vi "Compression_Simulation_Get Target Measurements.vi"(7 "Pout at Pin (dBm)":dbl, 8 "PAEs in":dbl[](array[numeric]), 9 "POUTs in":dbl[](array[numeric]), 10 "GAINs in":dbl[](array[numeric]), 11 "PINs in":dbl[](array[numeric])) -> (1 "PAE@Pin":dbl, 2 "Gain@Pin":dbl, 3 "Pout@Pin":dbl)   [LabVIEW 2023]
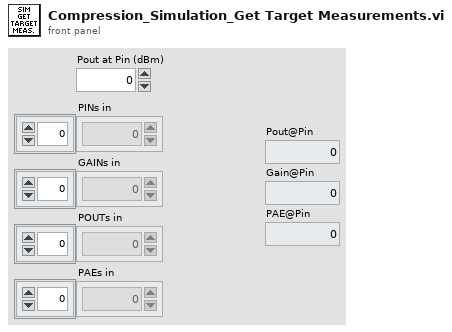
[diagram p1: front panel]
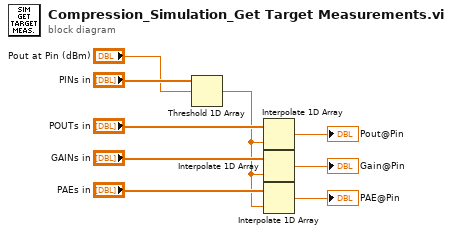
[diagram p0: block diagram]
diagram:
  n1 = Threshold 1D Array(2:"Pout at Pin (dBm)", 3:"PINs in") -> (0:w2:dbl)  [unwired: 1 in]
  n2 = Interpolate 1D Array(1:w2, 2:"POUTs in") -> (0:→"Pout@Pin":dbl)
  n3 = Interpolate 1D Array(1:w2, 2:"GAINs in") -> (0:→"Gain@Pin":dbl)
  n4 = Interpolate 1D Array(1:w2, 2:"PAEs in") -> (0:→"PAE@Pin":dbl)
